vi "list_toplevel_configurations.vi"(8 "error in (no error)":errorcluster, 10 "folder path of main configuration files":path, 11 "tree ref":refnum<vi>) -> (0 "error out":errorcluster)   [LabVIEW 2010]
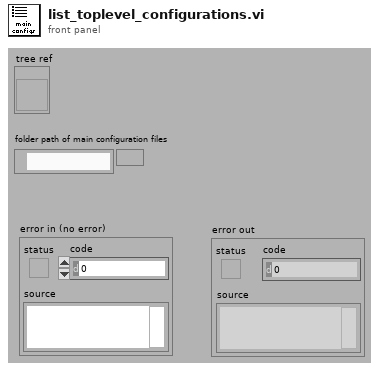
[diagram p1: front panel]
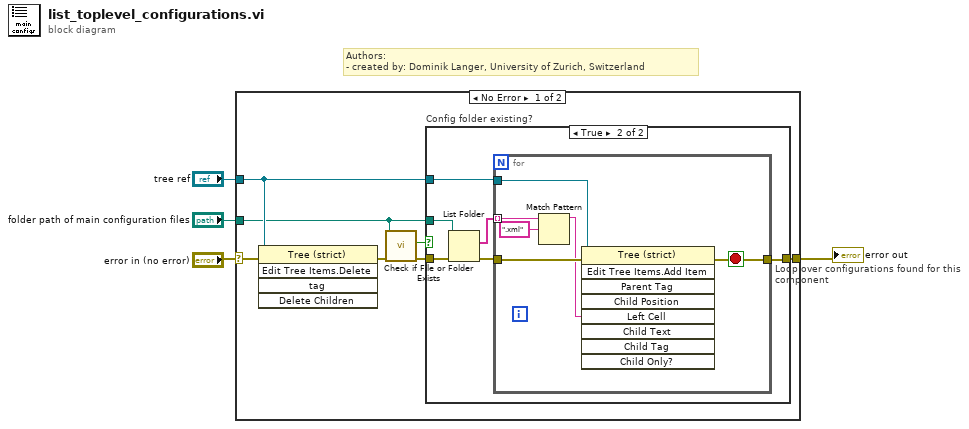
[diagram p0: block diagram]
diagram:
  # "Authors: \n- created by: Dominik Langer, University of Zurich, Switzerland"
  n1 = case shown="No Error" "error in (no error)" {
    selector: "error in (no error)" -> [w11 w25]
    tunnel: "tree ref" -> [w9 _]
    tunnel: [w10 w25] -> w2
    tunnel: "folder path of main configuration files" -> [w5 _]
    frame No Error {
      n2 = invoke on="Invoke Node" class="Tree (strict)" method="Edit Tree Items.Delete"(reference=w9, error in=w11) -> (error out=w6:errorcluster)  [unwired: 3 in, 4 out]
      n3 = call <vilib>:"Check if File or Folder Exists.vi"("error in (no error)"=w6, "path"=w5) -> ("error out"=w8:errorcluster, "file or folder exists?"=w7:bool)  [unwired: 8 out]
      n4 = case "Config folder existing?" shown="True" w7 {
        tunnel: [w12 w17] -> w10
        tunnel: w9 -> [_ w16]
        tunnel: w8 -> [w12 w14]
        tunnel: w5 -> [_ w13]
        frame False {
        }
        frame True {
          n5 = List Folder(path=w13, error in=w14) -> (filenames=w15:string[], error out=w18:errorcluster)  [unwired: 4 out]
          n6 = for "Loop over configurations found for this component" {
            tunnel: w15 -> [w23] mode=indexing
            tunnel: w16 -> [w20]
            tunnel: w18 -> [w24]
            tunnel: [w19] -> w17
            stop <- w19 stop-if-true
            n7 = Match Pattern(string=w23, regular expression=".xml") -> (before substring=w21:string)  [unwired: 4 out]
            n8 = invoke on="Invoke Node" class="Tree (strict)" method="Edit Tree Items.Add Item"(reference=w20, error in=w24, "Left Cell"=w21) -> (error out=w19:errorcluster)  [unwired: 6 in, 8 out]
          }
        }
      }
    }
    frame Error {
    }
  }
  "error out" <- w2
